vi "test Deadlock Wait and Conclude.vi"(8 "error in":errorcluster) -> (0 "error out":errorcluster)   [LabVIEW 2020, in "ase.test.lvlib"]
uses:
  ase.test.lvlib
  <vilib>/addons/_JKI Toolkits/Caraya/classes/Test/Test.lvclass
  ase/ase/ase.lvclass
  <vilib>/addons/_JKI Toolkits/Caraya/classes/Assert/Assert.lvclass
  <vilib>/addons/_JKI Toolkits/Caraya/classes/Assert/Assert Almost Equal_Float.vi
  8470fbbf-866f-49e0-b1d3-358e7939692e.vi
  b0138b9c-6e41-4bb4-8eec-ebe8f066c01e.vi
  <vilib>/addons/_JKI Toolkits/Caraya/classes/Assert/Assert Less_Variant.vi
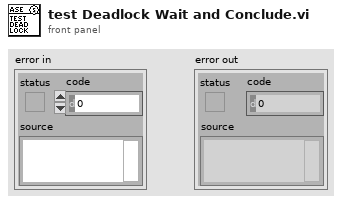
[diagram p1: front panel]
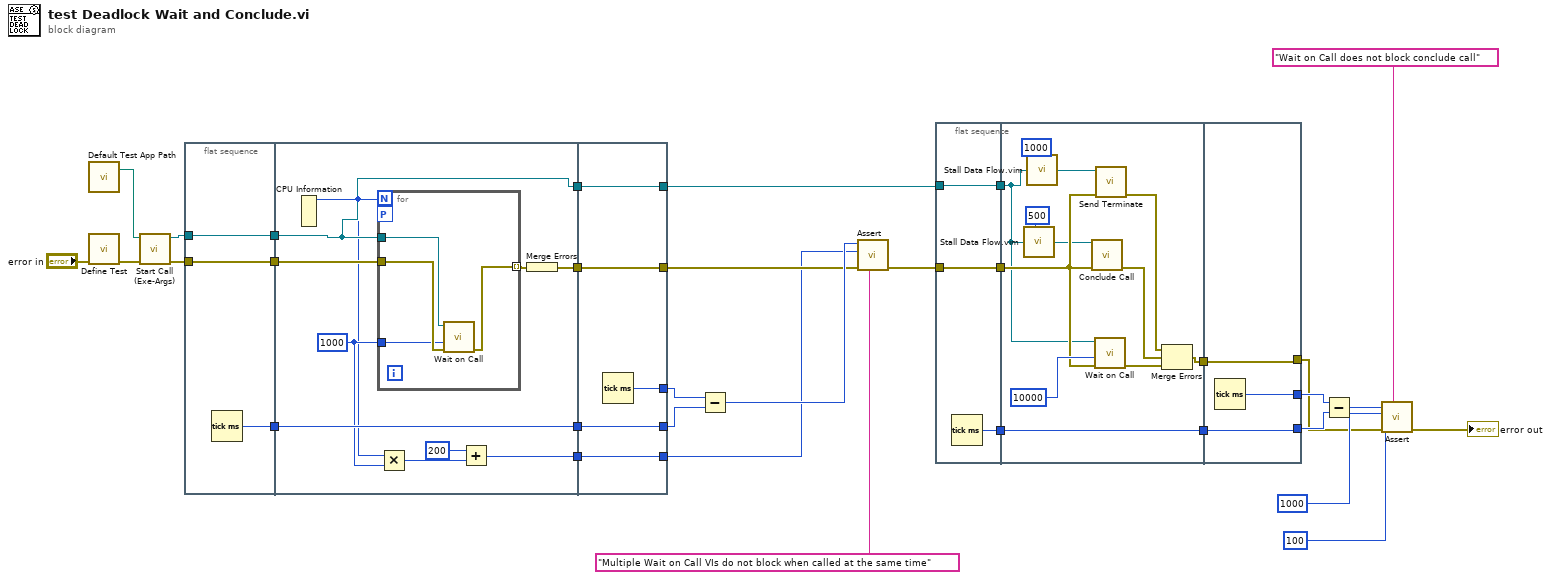
[diagram p0: block diagram]
diagram:
  n1 = call "Default Test App Path.vi"() -> ("Exe Path With Extention"=w1:path)  [unwired: 2 in, 1 out]
  n2 = call <vilib>:"Define Test.vi"("error in (no error)"="error in") -> ("error out"=w32:errorcluster)  [unwired: 9 in, 1 out]
  n3 = call "Start Call (Exe-Args).vi"("error in"=w32, "Executable Path"=w1) -> ("error out"=w31:errorcluster, "New ASE Handle"=w30:refnum<class "ase.lvclass">)  [unwired: 8 in]
  n4 = flat-sequence {
    tunnel: w30 -> [w35]
    tunnel: w31 -> [w36]
    tunnel: [w36] -> w29
    tunnel: [w35] -> w28
    tunnel: [w34] -> w26
    tunnel: w29 -> [w46]
    tunnel: w28 -> [w42]
    tunnel: [w45] -> w27
    tunnel: w26 -> [w45]
    tunnel: [w43] -> w7
    tunnel: [w42] -> w4
    tunnel: [w38] -> w3
    tunnel: w27 -> [w55]
    tunnel: [w55] -> w24
    tunnel: [w54] -> w25
    tunnel: [w53] -> w8
    tunnel: w7 -> [w53]
    tunnel: [w52] -> w5
    tunnel: w4 -> [w52]
    tunnel: [w51] -> w2
    tunnel: w3 -> [w51]
    frame #0 {
      n5 = Tick Count (ms)() -> (millisecond timer value=w34:u32)
    }
    frame #1 {
      w41 = 1000 ("Timeout (ms)")
      n6 = CPU Information() -> (4:w40:i32)  [unwired: 3 out]
      n7 = for {
        N: w40 -> [_]
        tunnel: w46 -> [w50]
        tunnel: w42 -> [w49]
        workers-P: _ -> [_]
        tunnel: [w48] -> w44 mode=indexing
        tunnel: w41 -> [w47]
        n8 = call "Wait on Call.vi"("error in"=w50, "Timeout (ms)"=w47, "ASE Handle"=w49) -> ("error out"=w48:errorcluster)  [unwired: 6 in, 2 out]
      }
      n9 = Multiply(x=w40, y=w41) -> (x*y=w39:i32)
      n10 = Add(x=200, y=w39) -> (x+y=w38:i32)
      n11 = Merge Errors(w44) -> (w43:errorcluster)
    }
    frame #2 {
      n12 = Tick Count (ms)() -> (millisecond timer value=w54:u32)
    }
  }
  n13 = Subtract(x=w25, y=w24) -> (x-y=w23:u32)
  n14 = call-poly <vilib>:"Assert.vi"("Label"="Multiple Wait on Call VIs do not block when called at the same time", "error in (no error)"=w8, "Y"=w2, "X"=w23) -> ("error out"=w21:errorcluster)  [unwired: 6 in, 1 out]
  n15 = flat-sequence {
    tunnel: w21 -> [w58]
    tunnel: [w58] -> w20
    tunnel: [w57] -> w19
    tunnel: [w56] -> w6
    tunnel: w5 -> [w56]
    tunnel: w20 -> [w64]
    tunnel: w19 -> [w65]
    tunnel: [w66] -> w18
    tunnel: [w65] -> w17
    tunnel: w6 -> [w61]
    tunnel: [w73] -> w12
    tunnel: w18 -> [w73]
    tunnel: [w72] -> w16
    tunnel: [w71] -> w15
    tunnel: w17 -> [w71]
    frame #0 {
      n16 = Tick Count (ms)() -> (millisecond timer value=w57:u32)
    }
    frame #1 {
      n17 = call "Stall Data Flow.vim"("value in"=w61, "milliseconds to wait"=u32 500) -> ("value out"=w60:refnum<class "ase.lvclass">)  [unwired: 1 out]
      n18 = call "Stall Data Flow.vim"("value in"=w61, "milliseconds to wait"=u32 1000) -> ("value out"=w59:refnum<class "ase.lvclass">)  [unwired: 1 out]
      n19 = call "Conclude Call.vi"("error in"=w64, "ASE Handle"=w60) -> ("error out"=w68:errorcluster)  [unwired: 7 in, 2 out]
      n20 = call "Wait on Call.vi"("error in"=w64, "Timeout (ms)"=10000, "ASE Handle"=w61) -> ("error out"=w67:errorcluster)  [unwired: 6 in, 2 out]
      n21 = call "Send Terminate.vi"("error in"=w64, "ASE Handle"=w59) -> ("error out"=w63:errorcluster)  [unwired: 7 in, 2 out]
      n22 = Merge Errors(w63, w68, w67) -> (w66:errorcluster)
    }
    frame #2 {
      n23 = Tick Count (ms)() -> (millisecond timer value=w72:u32)
    }
  }
  n24 = Subtract(x=w16, y=w15) -> (x-y=w14:u32)
  n25 = call-poly <vilib>:"Assert.vi"("Label"="Wait on Call does not block conclude call", "error in (no error)"=w12, "Tolerance"=100 ("Y"), "Y"=1000, "X"=w14) -> ("error out"=→"error out":errorcluster)  [unwired: 5 in, 1 out]
